vi "CheckIfAttrLocked.vi"(0 "reference in":refnum<class "G#BaseClass2.lvclass">, 5 "error in (no error)":errorcluster) -> (14 "reference out":refnum<class "G#BaseClass2.lvclass">, 15 "locked":bool, 19 "error out":errorcluster)   [LabVIEW 2010, in "G#BaseClass2.lvclass"]
uses:
  G#BaseClass2.lvclass
  G#BaseClass2.lvclass/G#BaseClass2.ctl
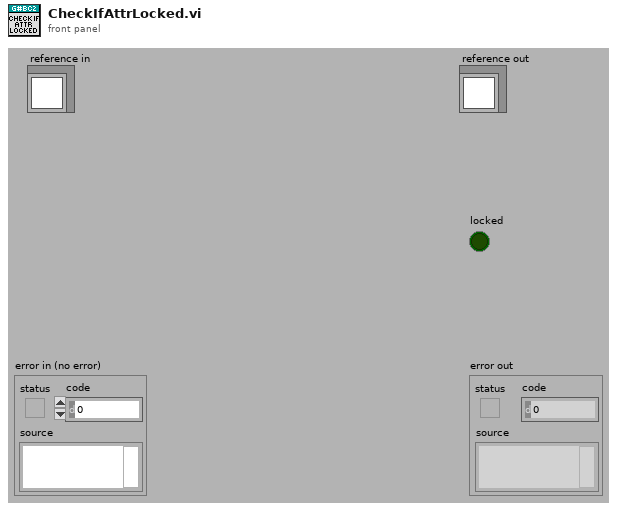
[diagram p1: front panel]
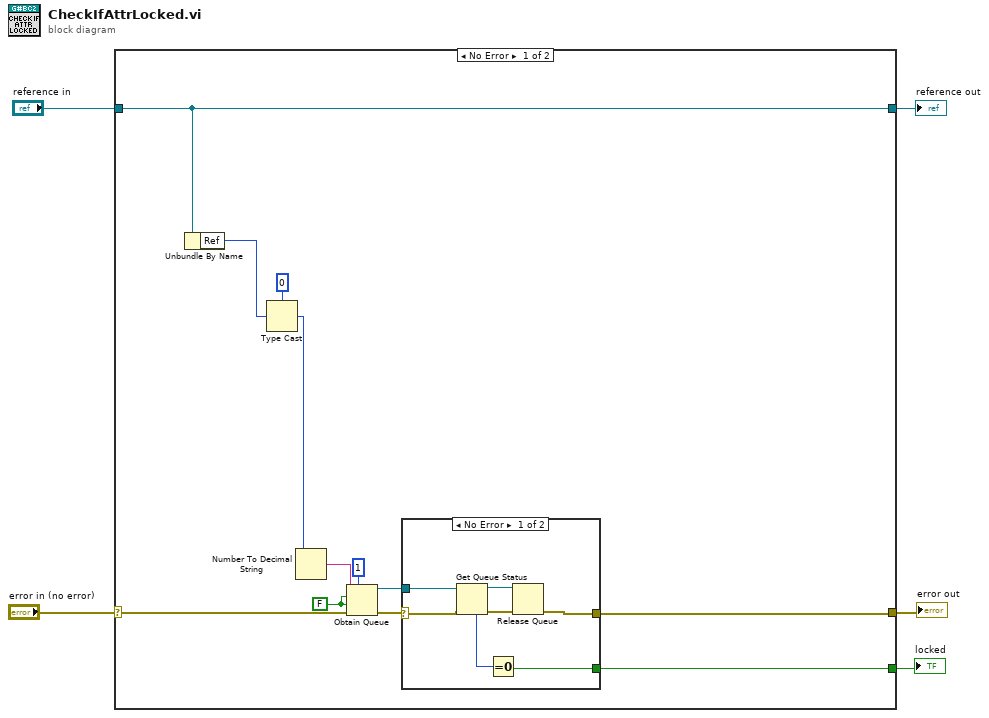
[diagram p0: block diagram]
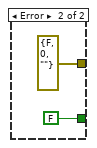
[diagram p2: hidden frame]
diagram:
  n1 = case shown="No Error" "error in (no error)" {
    selector: "error in (no error)" -> [w12 w28]
    tunnel: [w8 w28] -> w4
    tunnel: [w17 w27] -> w2
    tunnel: "reference in" -> [w17 w27]
    tunnel: [w6 _] -> w1
    frame No Error {
      w15 = FALSE ("create if not found? (T)")
      n2 = Unbundle By Name(w17) -> ("Ref"=w11:u32)
      n3 = Type Cast(type=u32 0, x=w11) -> (*(type *) &x=w10:u32)
      n4 = Number To Decimal String(number=w10) -> (decimal integer string=w16:string)  [unwired: 1 in]
      n5 = Obtain Queue(max queue size (-1, unlimited)=1, name (unnamed)=w16, element data type=w15, create if not found? (T)=w15, error in (no error)=w12) -> (queue out=w9:refnum<queue>, error out=w7:errorcluster)  [unwired: 1 out]
      n6 = case shown="No Error" w7 {
        selector: w7 -> [w20 _]
        tunnel: w9 -> [w24 _]
        tunnel: [w23 errorcluster {"status"=FALSE, "code"=0, "source"=""} ("error out")] -> w8
        tunnel: [w19 FALSE] -> w6
        frame No Error {
          n7 = Get Queue Status(queue=w24, error in (no error)=w20) -> (queue out=w21:refnum<queue>, error out=w22:errorcluster, # elements in queue=w18:i32)  [unwired: 1 in, 5 out]
          n8 = Equal To 0?(x=w18) -> (x = 0?=w19:bool)
          n9 = Release Queue(queue=w21, error in (no error)=w22) -> (error out=w23:errorcluster)  [unwired: 1 in, 2 out]
        }
        frame Error {
        }
      }
    }
    frame Error {
    }
  }
  "error out" <- w4
  "reference out" <- w2
  "locked" <- w1
